vi "sub parse sound.vi"(8 "error in":errorcluster, 11 "sound string":string) -> (0 "error out":errorcluster, 3 "sound":string)   [LabVIEW 2018, in "Data Parser.lvclass"]
uses:
  Data Parser.lvclass
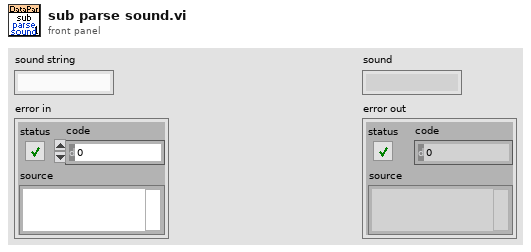
[diagram p1: front panel]
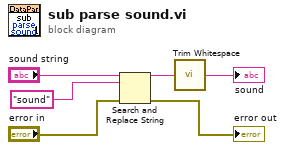
[diagram p0: block diagram]
diagram:
  n1 = Search and Replace String(input string="sound string", search string="sound", error in="error in") -> (result string=w2:string, error out=→"error out":errorcluster)  [unwired: 5 in, 2 out]
  n2 = call <vilib>:"Trim Whitespace.vi"("string"=w2) -> ("trimmed string"=→"sound":string)  [unwired: 1 in]
